vi "Replace Template Async Ref.vi"(6 "VI Ref Const Label":string="Static VI Reference", 8 "error in (no error)":errorcluster, 10 "Path to Desired Async VI":path, 11 "Path to RT Driver VI":path) -> (0 "error out":errorcluster)   [LabVIEW 2015]
doc: "This VI allows you to set the path to a static VI reference based on the name of the VI reference constant."
uses:
  <vilib>/Utility/traverseref.llb/TRef TravTarget.ctl
  <vilib>/Utility/traverseref.llb/VI Scripting - Traverse.lvlib
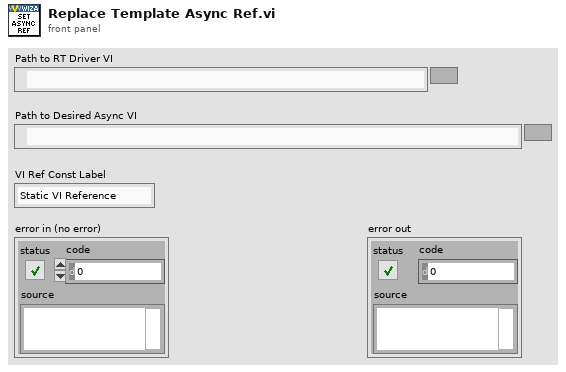
[diagram p1: front panel]
types:
  T1 = typedef "TRef TravTarget.ctl" = enum16{"FP", "BD", "Other"}
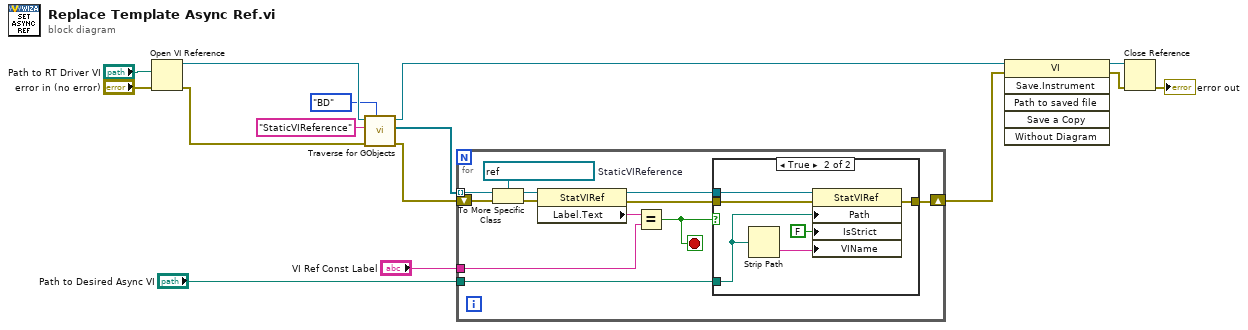
[diagram p0: block diagram]
diagram:
  n1 = Open VI Reference(vi path="Path to RT Driver VI", error in (no error)="error in (no error)") -> (vi reference=w7:refnum<vi>, error out=w8:errorcluster)  [unwired: 4 in]
  n2 = call <vilib>:"Traverse for GObjects.vi"("Traverse Target"=TRef_TravTarget."BD", "error in (no error)"=w8, "Class Name"="StaticVIReference", "VI Refnum"=w7) -> ("error out"=w5:errorcluster, "References"=w4:refnum<vi>[], "dup VI Refnum"=w9:refnum<vi>)  [unwired: 4 in, 1 out]
  n3 = for {
    tunnel: w4 -> [w27] mode=indexing
    shift-right: [w17] -> w13
    shift-left: w5 -> [w25]
    tunnel: "VI Ref Const Label" -> [w21]
    tunnel: "Path to Desired Async VI" -> [w18]
    stop <- w16 stop-if-true
    w26 = refnum<vi> refnum  # StaticVIReference
    n4 = To More Specific Class(target class=w26, reference=w27, error in=w25) -> (specific class reference=w24:refnum<vi>, error out=w23:errorcluster)
    n5 = property class="StatVIRef"(reference=w24, error in=w23) -> (reference out=w20:refnum<vi>, error out=w19:errorcluster, "Label.Text"=w22:string)
    n6 = Equal?(x=w22, y=w21) -> (x = y?=w16:bool)
    n7 = case shown="True" w16 {
      tunnel: w20 -> [_ w33]
      tunnel: w19 -> [w28 w32]
      tunnel: w18 -> [_ w31]
      tunnel: [w28 w34] -> w17
      frame False {
      }
      frame True {
        n8 = Strip Path(path=w31) -> (name=w30:string)  [unwired: 1 out]
        n9 = property class="StatVIRef"(reference=w33, error in=w32, "Path"=w31, "IsStrict"=FALSE ("Is Strict"), "VIName"=w30) -> (error out=w34:errorcluster)  [unwired: 1 out]
      }
    }
  }
  n10 = invoke class="VI" method="Save.Instrument"(reference=w9, error in=w13) -> (reference out=w10:refnum<vi>, error out=w11:errorcluster)  [unwired: 4 in, 4 out]
  n11 = Close Reference(reference=w10, error in (no error)=w11) -> (error out=→"error out":errorcluster)
